vi "ADS Load Model.vi"(8 "error in (no error)":errorcluster, 10 "ref in":u64, 11 "Model Path":path) -> (0 "error out":errorcluster, 2 "ref out":u64, 3 "success":i32)   [LabVIEW 2024]
uses:
  dependencies_dll_release/TCV_Lib.dll
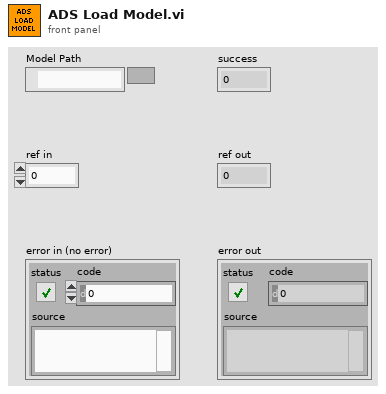
[diagram p1: front panel]
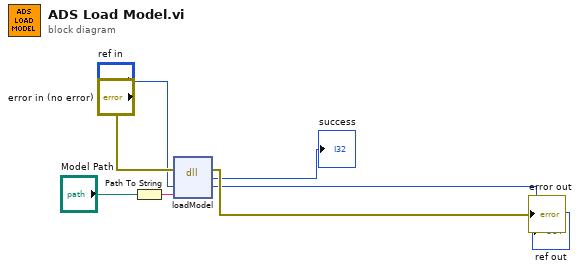
[diagram p0: block diagram]
diagram:
  n1 = Path To String(path="Model Path") -> (string=w2:string)
  n2 = dll-call lib="D:/labviewTestTCVdll/TransformCV-LabVIEW/Test/dependencies_dll_release/TCV_Lib.dll" fn="loadModel"(error in="error in (no error)", "ref"="ref in", "path"=w2) -> (error out=→"error out":errorcluster, "success"=→"success":i32, "ref"=→"ref out":u64)  [unwired: 3 in, 1 out]
